vi "All object detection.vi"() -> ()   [LabVIEW 2018]
panel:
  out "error out":errorcluster
  out "Image":T1(plugin-control)
  out "Frame Rate":dbl
  in  "stop":bool
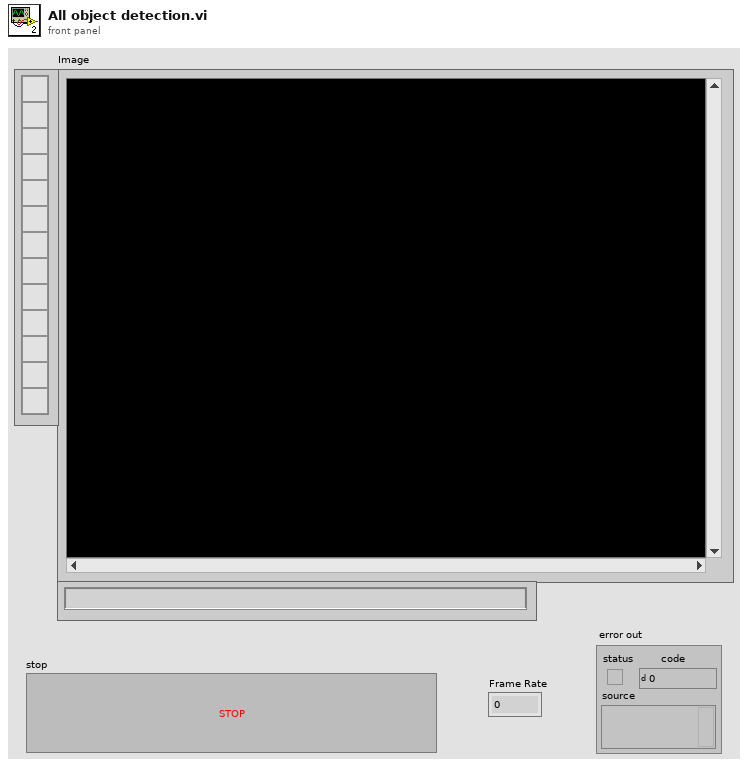
[diagram p1: front panel]
types:
  T1 = typedef "IMAQ Image.ctl" = refnum<image>
  T2 = cluster{"Global Rectangle":cluster{"x1Left":i32, "y1Top":i32, "x2Right":i32, "y2Bottom":i32}, "Centroid":cluster{"x":sgl, "y":sgl}, "Object Size":u32, "Score":dbl}[]
  T3 = cluster{"Shape Report (Shape Matching 1)[0]":cluster{"Global Rectangle":cluster{"x1Left":i32, "y1Top":i32, "x2Right":i32, "y2Bottom":i32}, "Centroid":cluster{"x":sgl, "y":sgl}, "Object Size":u32, "Score":dbl}, "Shape Report (Shape Matching 1)[1]":cluster{"Global Rectangle":cluster{"x1Left":i32, "y1Top":i32, "x2Right":i32, "y2Bottom":i32}, "Centroid":cluster{"x":sgl, "y":sgl}, "Object Size":u32, "Score":dbl}, "Shape Report (Shape Matching 1)[2]":cluster{"Global Rectangle":cluster{"x1Left":i32, "y1Top":i32, "x2Right":i32, "y2Bottom":i32}, "Centroid":cluster{"x":sgl, "y":sgl}, "Object Size":u32, "Score":dbl}, "Shape Report (Shape Matching 1)[3]":cluster{"Global Rectangle":cluster{"x1Left":i32, "y1Top":i32, "x2Right":i32, "y2Bottom":i32}, "Centroid":cluster{"x":sgl, "y":sgl}, "Object Size":u32, "Score":dbl}, "Shape Report (Shape Matching 1)[4]":cluster{"Global Rectangle":cluster{"x1Left":i32, "y1Top":i32, "x2Right":i32, "y2Bottom":i32}, "Centroid":cluster{"x":sgl, "y":sgl}, "Object Size":u32, "Score":dbl}, "Shape Report (Shape Matching 1)[5]":cluster{"Global Rectangle":cluster{"x1Left":i32, "y1Top":i32, "x2Right":i32, "y2Bottom":i32}, "Centroid":cluster{"x":sgl, "y":sgl}, "Object Size":u32, "Score":dbl}, "Shape Report (Shape Matching 1)[6]":cluster{"Global Rectangle":cluster{"x1Left":i32, "y1Top":i32, "x2Right":i32, "y2Bottom":i32}, "Centroid":cluster{"x":sgl, "y":sgl}, "Object Size":u32, "Score":dbl}, "Shape Report (Shape Matching 1)[7]":cluster{"Global Rectangle":cluster{"x1Left":i32, "y1Top":i32, "x2Right":i32, "y2Bottom":i32}, "Centroid":cluster{"x":sgl, "y":sgl}, "Object Size":u32, "Score":dbl}, "Shape Report (Shape Matching 1)[8]":cluster{"Global Rectangle":cluster{"x1Left":i32, "y1Top":i32, "x2Right":i32, "y2Bottom":i32}, "Centroid":cluster{"x":sgl, "y":sgl}, "Object Size":u32, "Score":dbl}}
  T4 = cluster{"Global Rectangle":cluster{"x1Left":i32, "y1Top":i32, "x2Right":i32, "y2Bottom":i32}, "Centroid":cluster{"x":sgl, "y":sgl}, "Object Size":u32, "Score":dbl}
  T5 = cluster{"x1Left":i32, "y1Top":i32, "x2Right":i32, "y2Bottom":i32}
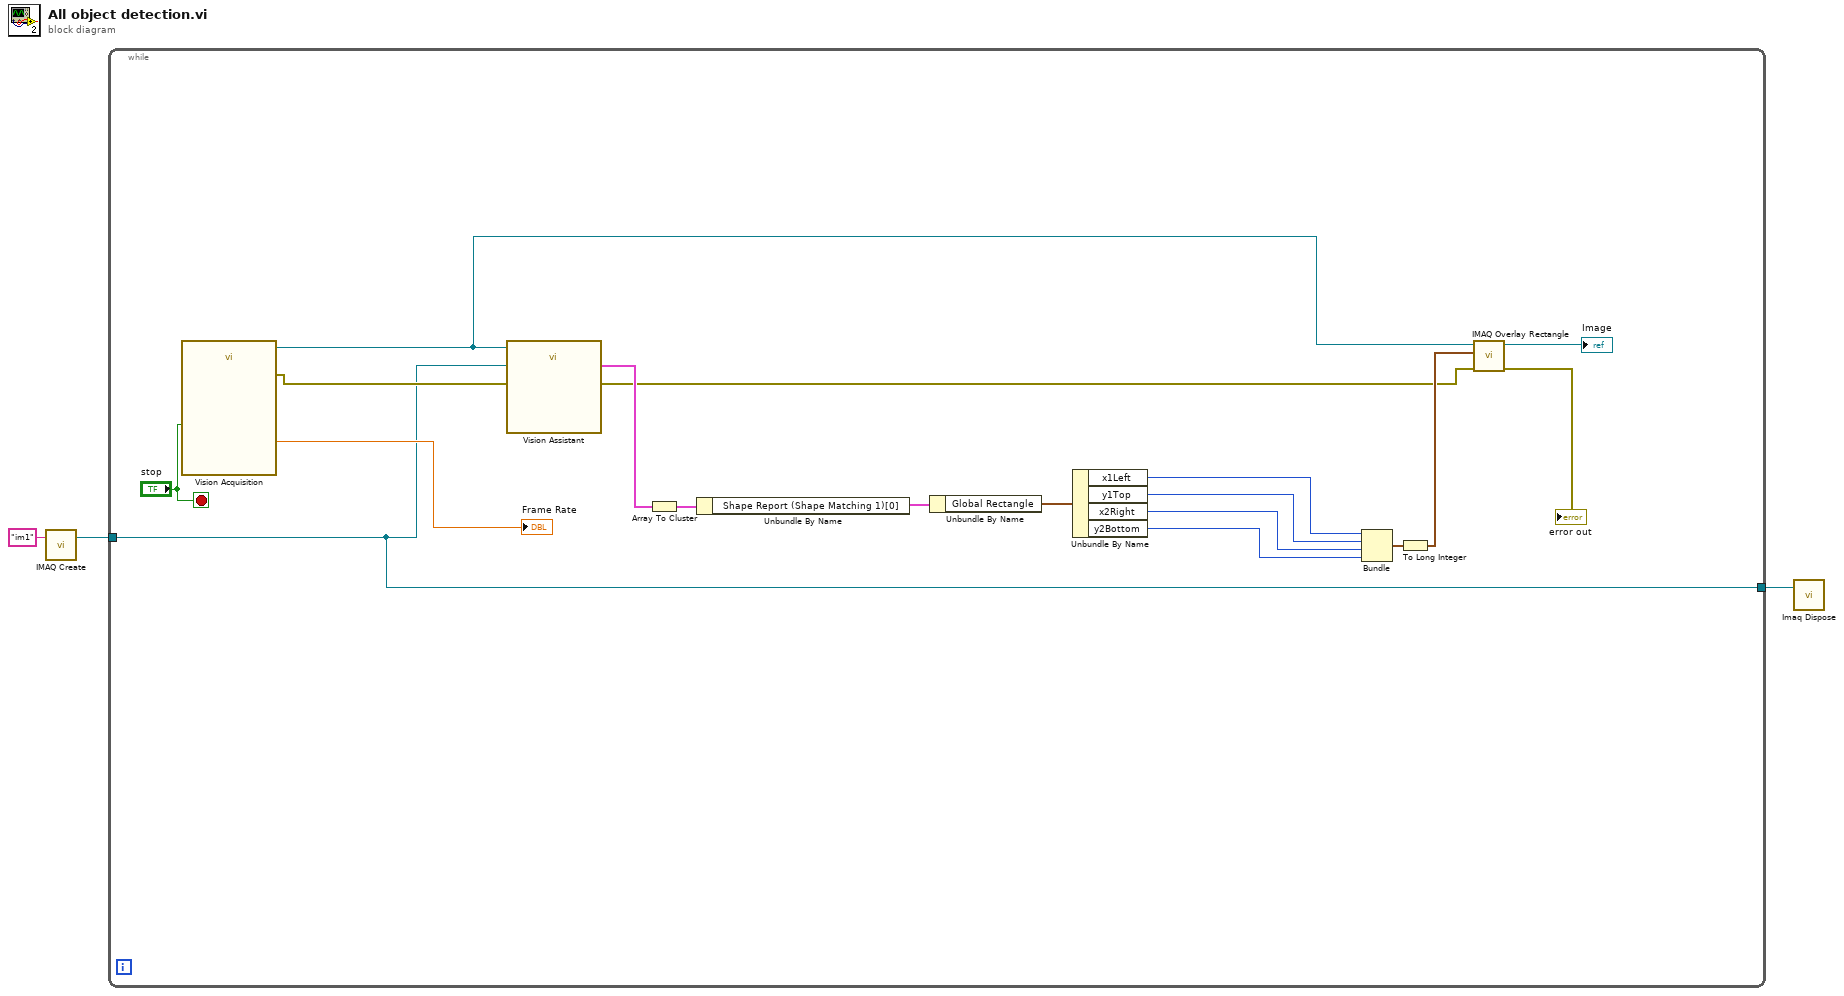
[diagram p0: block diagram]
diagram:
  n1 = call "IMAQ Create"("Image Name"="im1") -> ("New Image"=w3:T1)  [unwired: 4 in, 1 out]
  n2 = while {
    tunnel: w3 -> [w4]
    tunnel: [w4] -> w1
    stop <- "stop" stop-if-true
    n3 = call "Vision Acquisition"("Stop (F)"="stop") -> ("Image Out"=w6:T1, "Frame Rate"=→"Frame Rate":dbl, "error out"=w9:errorcluster)  [unwired: 23 in, 1 out]
    n4 = call "Vision Assistant"("Image In"=w6, "Image Dst"=w4, "error in"=w9) -> ("Shape Report (Shape Matching 1)"=w18:T2, "error out"=w8:errorcluster)  [unwired: 20 in, 3 out]
    n5 = Array To Cluster(array=w18) -> (cluster=w19:T3)
    n6 = Unbundle By Name(w19) -> ("Shape Report (Shape Matching 1)[0]"=w17:T4)
    n7 = Unbundle By Name(w17) -> ("Global Rectangle"=w16:T5)
    n8 = Unbundle By Name(w16) -> ("x1Left"=w15:i32, "y1Top"=w14:i32, "x2Right"=w13:i32, "y2Bottom"=w12:i32)
    n9 = Bundle("x1Left"=w15, "y1Top"=w14, "x2Right"=w13, "y2Bottom"=w12) -> (w11:T5)  [unwired: 1 in]
    n10 = To Long Integer(number=w11) -> (32bit integer=w10:T5)
    n11 = call "IMAQ Overlay Rectangle"("error in (no error)"=w8, "Rectangle"=w10, "Image"=w6) -> ("error out"=→"error out":errorcluster, "Image Out"=→"Image":T1)  [unwired: 7 in]
  }
  n12 = call "Imaq Dispose"("Image"=w1) -> ()  [unwired: 5 in, 1 out]
